vi "LED blink.vi"() -> ()   [LabVIEW 2011]
panel:
  in  "stop":bool
  out "Boolean":bool
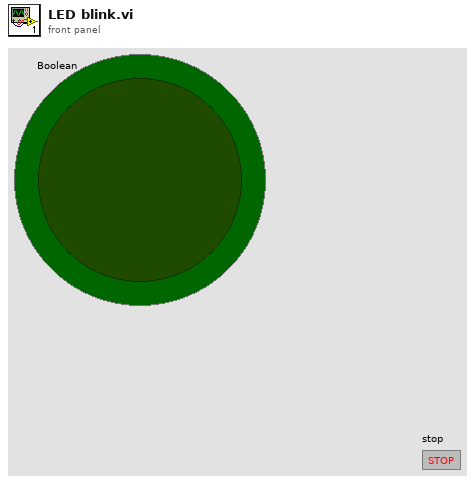
[diagram p1: front panel]
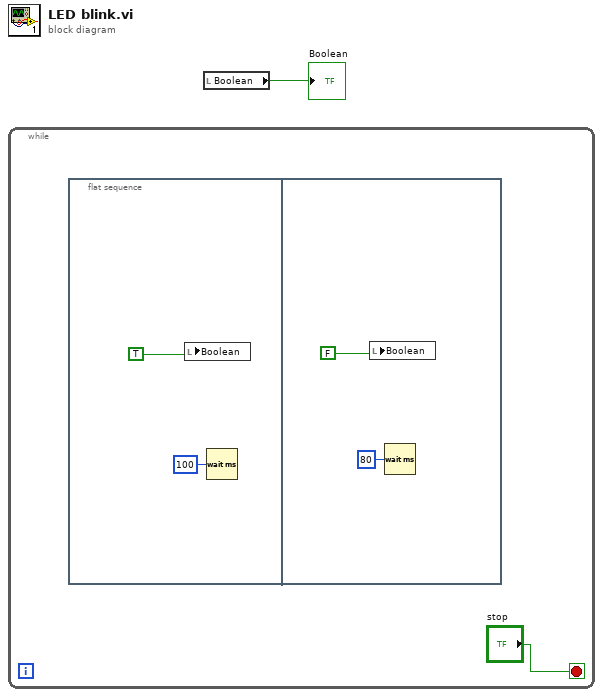
[diagram p0: block diagram]
diagram:
  n1 = while {
    stop <- "stop" stop-if-true
    n2 = flat-sequence {
      frame #0 {
        n3 = local write "Boolean"(TRUE) -> ()
        n4 = Wait (ms)(milliseconds to wait=u32 100) -> ()  [unwired: 1 out]
      }
      frame #1 {
        n5 = local write "Boolean"(FALSE) -> ()
        n6 = Wait (ms)(milliseconds to wait=u32 80) -> ()  [unwired: 1 out]
      }
    }
  }
  n7 = local read "Boolean"() -> (→"Boolean":bool)
